vi "Load X minus Y Delta.vi"(7 "Reinit":bool, 8 "error in (no error)":errorcluster, 9 "Y":i64, 10 "X":i64, 11 "Stats_I64_CIF_U in":refnum<class "Stats_I64_CIF_U.lvclass">) -> (0 "error out":errorcluster, 3 "Stats_I64_CIF_U out":refnum<class "Stats_I64_CIF_U.lvclass">)   [LabVIEW 2021, in "Stats_CIF_U.lvlib" / "Stats_I64_CIF_U.lvclass"]
doc: "Load a new data value into the statistics class. The new value will be calculated by subracting the X value from the Y value. This VI is useful for benchmarking where a timestamp is taken before and after a function."
uses:
  Stats_I64_CIF_U.lvclass
  Stats_I64_CIF_U.lvclass/Stats_I64_CIF_U.ctl
  dfabcf33-0dbc-4041-80a5-3dc0c86d2989.vi
  dfabcf33-0dbc-4041-80a5-3dc0c86d2989.vi/9eb60a9a-770f-4d2d-8b3f-8465c267ecc9.vi
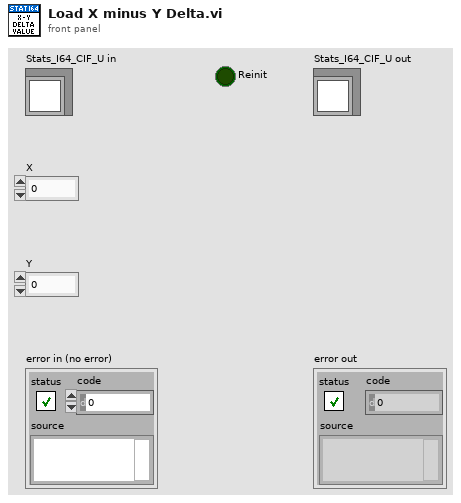
[diagram p1: front panel]
types:
  T1 = typedef "Stats_CIF_U.lvlib/I64 Stat Data.ctl" = cluster{"Last Value":i64, "Max":i64, "Min":i64, "Common ":T2}
  T2 = typedef "Stats_CIF_U.lvlib/Common Stat Data.ctl" = cluster{"Iteration":u32, "Max History":i32, "Average":dbl}
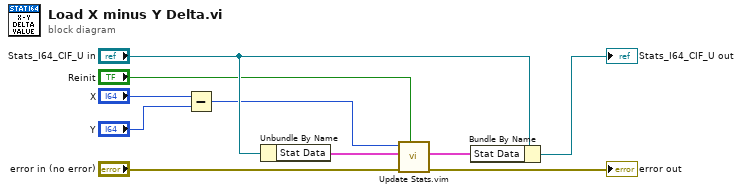
[diagram p0: block diagram]
diagram:
  n1 = Subtract(x="X", y="Y") -> (x-y=w1:i64)
  n2 = Unbundle By Name("Stats_I64_CIF_U in") -> ("Stat Data"=w8:T1)
  n3 = call "Update Stats.vim"("Reinit"="Reinit", "error in"="error in (no error)", "Stat Data In"=w8, "New Value"=w1) -> ("error out"=→"error out":errorcluster, "Stat Data Out"=w7:T1)  [unwired: 6 in]
  n4 = Bundle By Name(cluster="Stats_I64_CIF_U in", "Stat Data"=w7) -> (→"Stats_I64_CIF_U out":refnum<class "Stats_I64_CIF_U.lvclass">)
